vi "Shunting yard algorithm.vi"(2 "error in (no error)":errorcluster, 3 "Infix Notation Data":T1) -> (0 "error out":errorcluster, 1 "Postfix Notation Data":T1)   [LabVIEW 2020]
uses:
  <vilib>/Utility/error.llb/Error Cluster From Error Code.vi
  <vilib>/ErrorRing/Error Ring.xnode
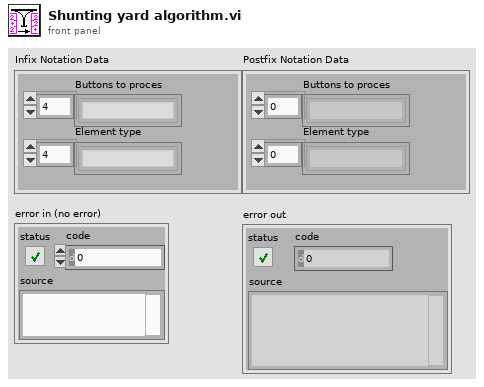
[diagram p1: front panel]
types:
  T1 = cluster{"Buttons to proces":string[], "Element type":string[]}
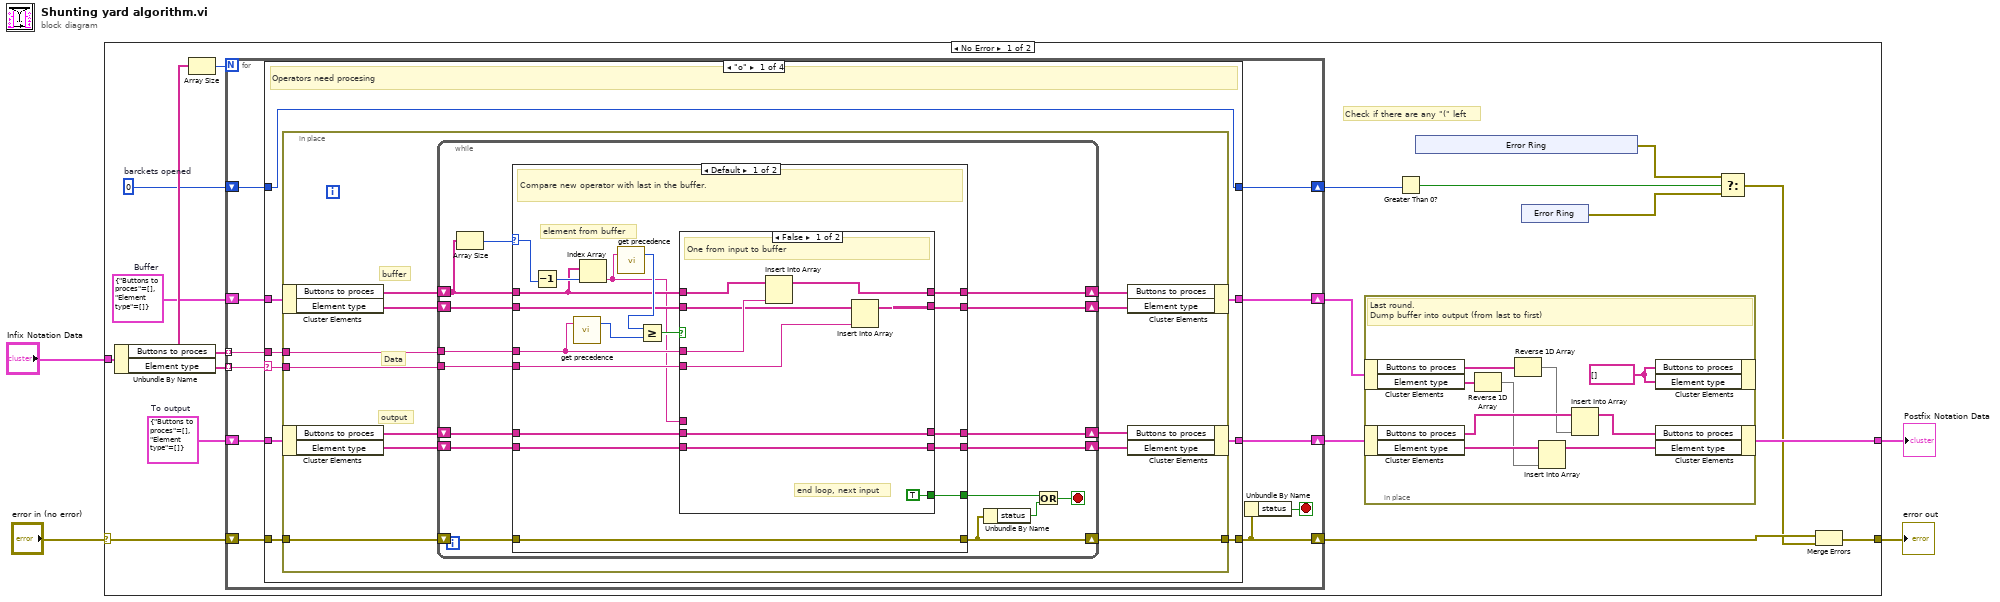
[diagram p0: block diagram]
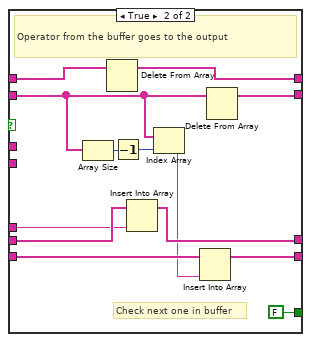
[diagram p2: hidden frame]
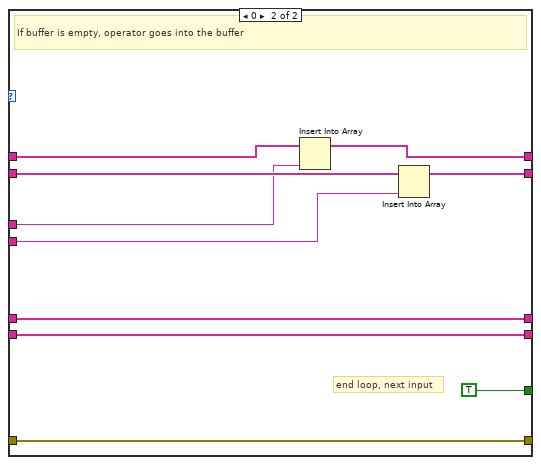
[diagram p3: hidden frame]
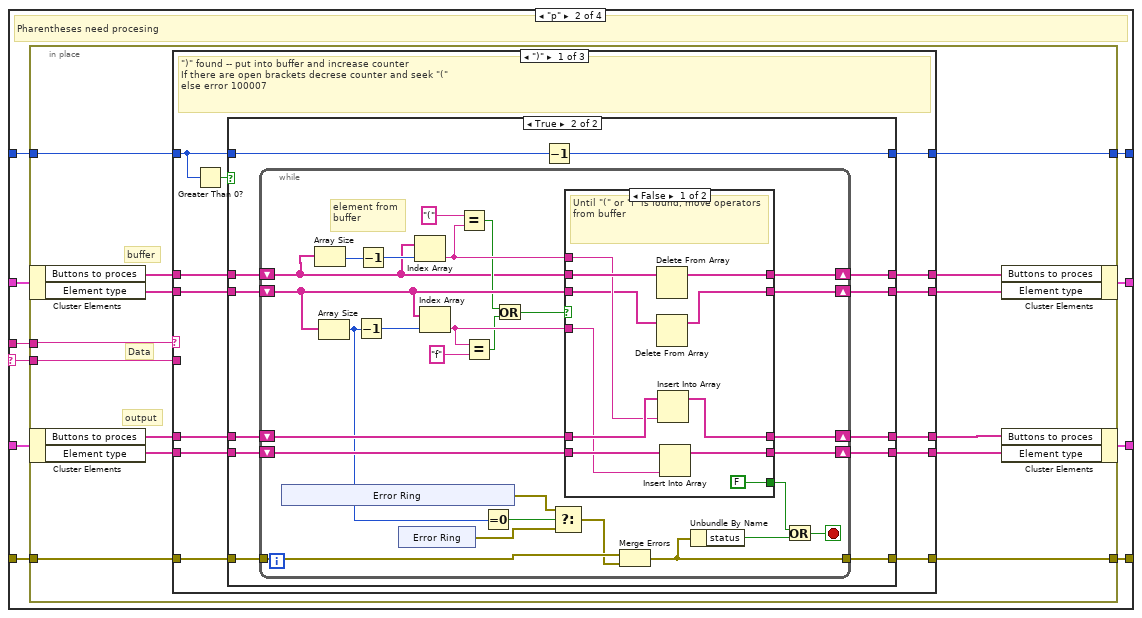
[diagram p4: hidden frame]
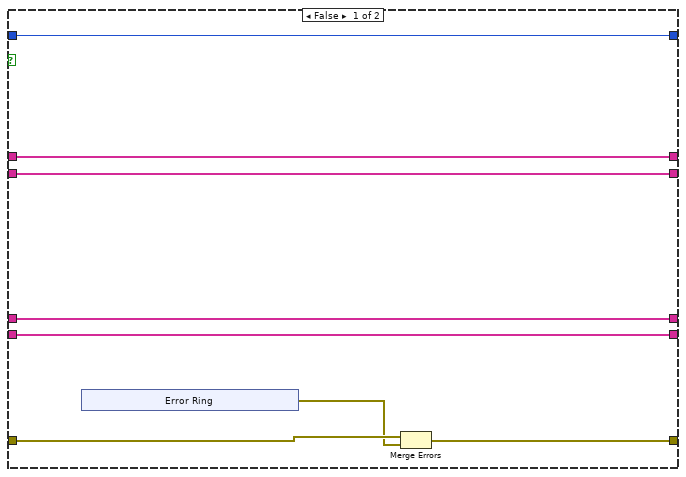
[diagram p5: hidden frame]
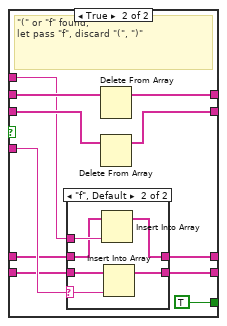
[diagram p6: hidden frame]
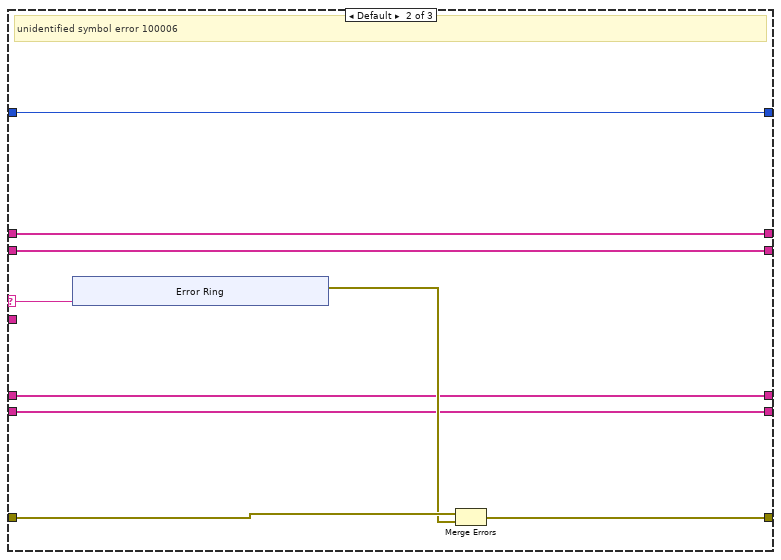
[diagram p8: hidden frame]
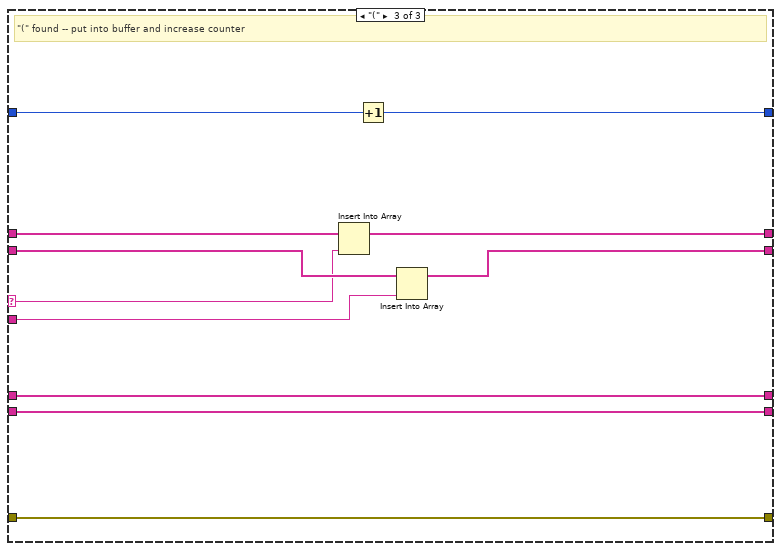
[diagram p9: hidden frame]
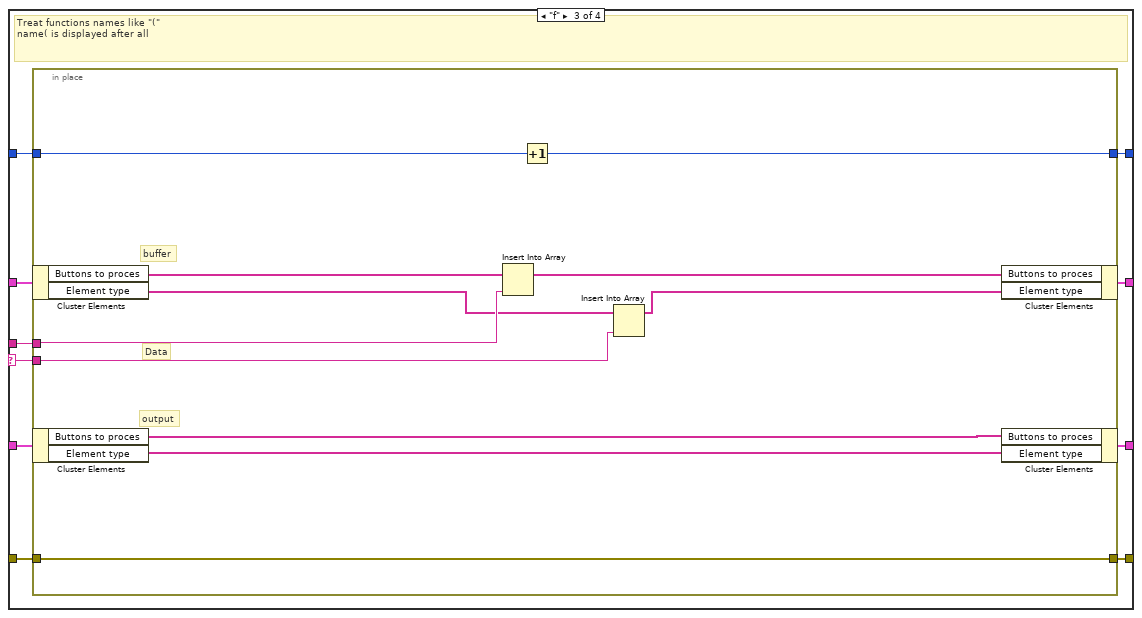
[diagram p10: hidden frame]
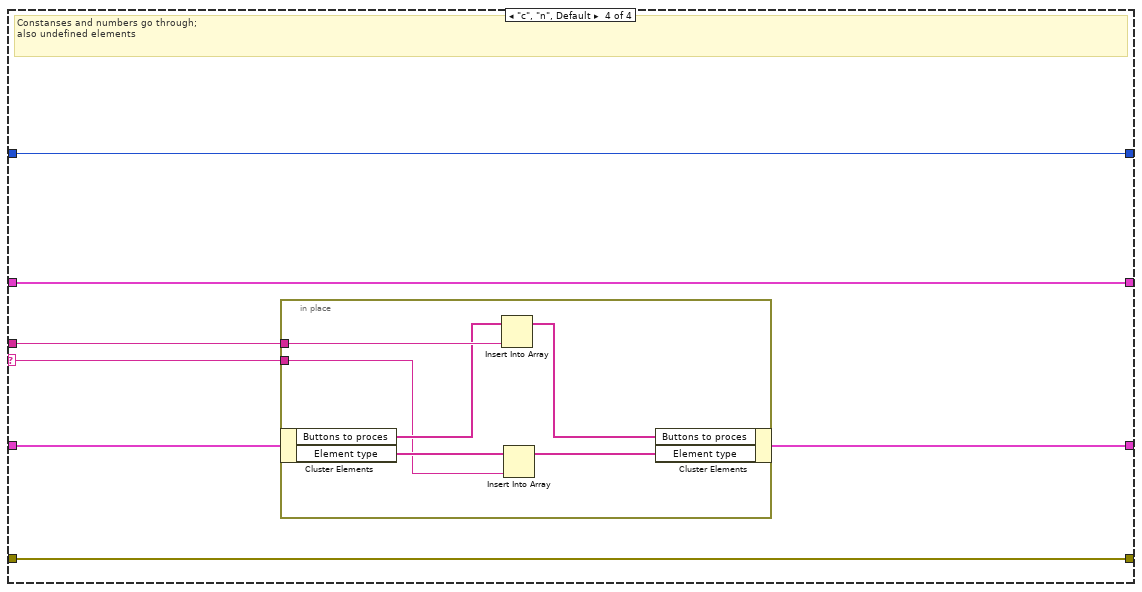
[diagram p11: hidden frame]
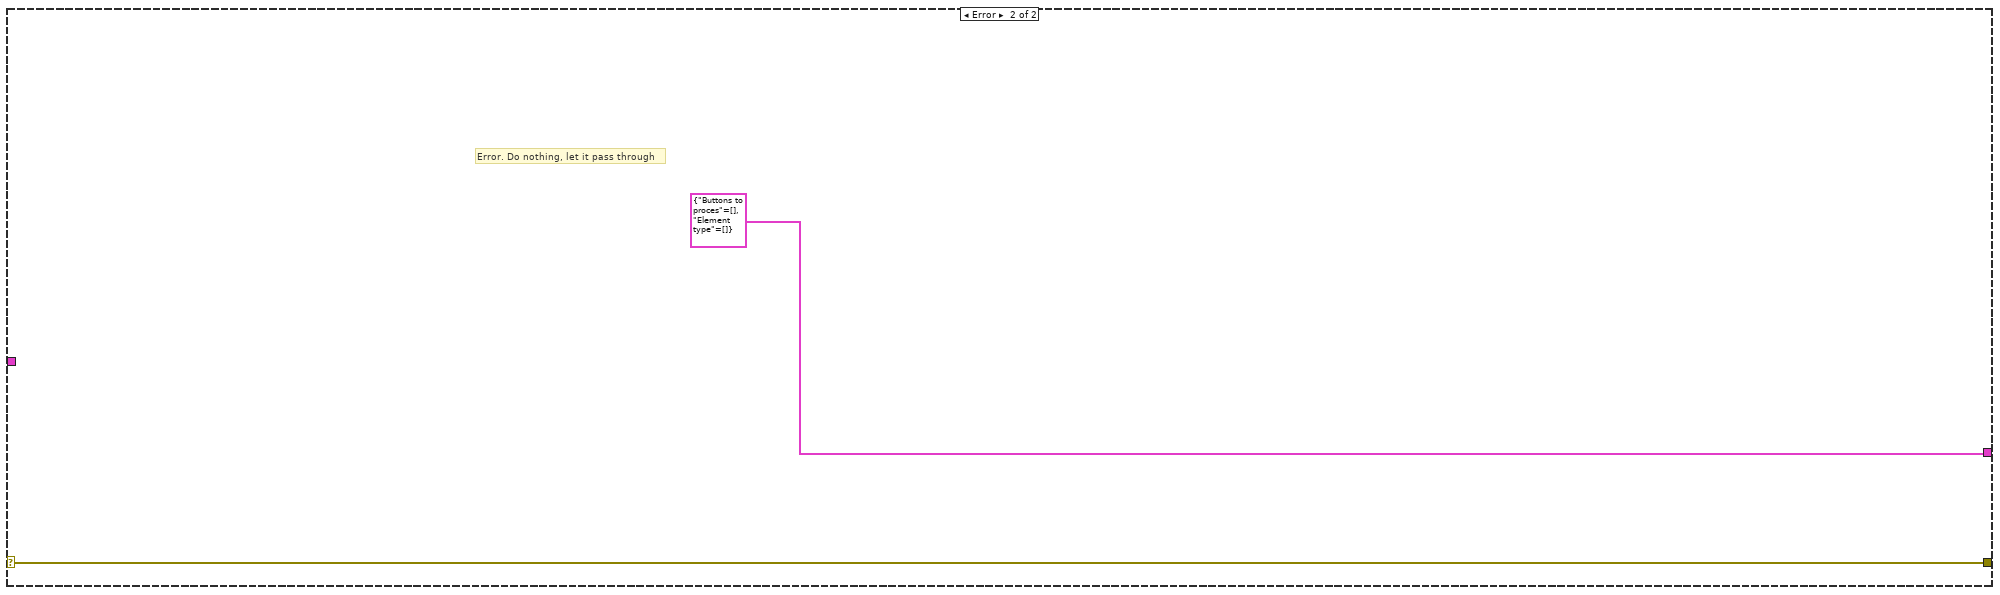
[diagram p12: hidden frame]
diagram:
  n1 = case shown="No Error" "error in (no error)" {
    selector: "error in (no error)" -> [w12 w324]
    tunnel: [w10 w324] -> w3
    tunnel: "Infix Notation Data" -> [w22 _]
    tunnel: [w14 T1 {"Buttons to proces"=[], "Element type"=[]} ("Input Data")] -> w1
    frame No Error {
      w11 = 0  # barckets opened
      w18 = T1 {"Buttons to proces"=[], "Element type"=[]}  # Buffer
      w19 = T1 {"Buttons to proces"=[], "Element type"=[]}  # To output
      # "Check if there are any \"(\" left"
      n2 = Unbundle By Name(w22) -> ("Buttons to proces"=w20:string[], "Element type"=w21:string[])
      n3 = Array Size(array=w20) -> (size(s)=w17:i32)
      n4 = for {
        N: w17 -> [_]
        tunnel: w21 -> [w43] mode=indexing
        tunnel: w20 -> [w44] mode=indexing
        shift-right: [w47] -> w15
        shift-left: w19 -> [w48]
        shift-right: [w45] -> w16
        shift-left: w18 -> [w46]
        shift-right: [w41] -> w13
        shift-left: w12 -> [w42]
        shift-right: [w38] -> w9
        shift-left: w11 -> [w39]
        stop <- w40 stop-if-true
        n5 = case shown="\"o\"" w43 {
          selector: w43 -> [w54 w142 w295 w314]
          tunnel: w48 -> [w57 w145 w298 w316]
          tunnel: [w52 w140 w293 w312] -> w47
          tunnel: w44 -> [w55 w143 w296 w315]
          tunnel: w46 -> [w56 w144 w297 w313]
          tunnel: [w53 w141 w294 w313] -> w45
          tunnel: w42 -> [w51 w139 w292 w311]
          tunnel: [w50 w138 w291 w311] -> w41
          tunnel: w39 -> [w49 w137 w290 w310]
          tunnel: [w49 w136 w289 w310] -> w38
          frame "o" {
            # "Operators need procesing"
            n6 = in-place {
              in-place-border: w55 -> [w63]
              in-place-border: w54 -> [w62]
              in-place-border: w51 -> [w69]
              in-place-border: [w68] -> w50
              # "Data"
              # "buffer"
              # "output"
              n7 = in-place-cluster #1(w56) -> ("Buttons to proces"=w61:string[], "Element type"=w60:string[])
              n8 = in-place-cluster #2(w57) -> ("Buttons to proces"=w65:string[], "Element type"=w64:string[])
              n9 = while {
                shift-right: [w73] -> w68
                shift-left: w69 -> [w74]
                shift-right: [w75] -> w58
                shift-left: w61 -> [w77]
                shift-right: [w78] -> w59
                shift-left: w60 -> [w79]
                shift-right: [w85] -> w67
                shift-left: w65 -> [w83]
                shift-right: [w84] -> w66
                shift-left: w64 -> [w82]
                tunnel: w63 -> [w81]
                tunnel: w62 -> [w80]
                stop <- w70 stop-if-true
                n10 = Array Size(array=w77) -> (size(s)=w76:i32)
                n11 = case shown="Default" w76 {
                  selector: w76 -> [w102 _]
                  tunnel: w83 -> [w94 w129]
                  tunnel: w82 -> [w89 w128]
                  tunnel: w77 -> [w96 w134]
                  tunnel: w79 -> [w98 w132]
                  tunnel: [w90 w128] -> w84
                  tunnel: [w91 w129] -> w85
                  tunnel: w80 -> [w92 w135]
                  tunnel: [w95 w133] -> w75
                  tunnel: [w97 w131] -> w78
                  tunnel: w81 -> [w93 w130]
                  tunnel: w74 -> [w87 w127]
                  tunnel: [w87 w127] -> w73
                  tunnel: [w86 TRUE] -> w71
                  frame Default {
                    # "element from buffer"
                    # "Compare new operator with last in the buffer."
                    n12 = Decrement(x=w102) -> (x-1=w103:i32)
                    n13 = call "get precedence.vi"("operator"=w93) -> ("Precedence"=w100:i32)  [unwired: 2 in]
                    n14 = Index Array(array=w96, index=w103) -> (element=w88:string)
                    n15 = call "get precedence.vi"("operator"=w88) -> ("Precedence"=w101:i32)  [unwired: 2 in]
                    n16 = Greater Or Equal?(x=w101, y=w100) -> (x >= y?=w99:bool)
                    n17 = case shown="False" w99 {
                      tunnel: w98 -> [w107 w115]
                      tunnel: [w104 w124] -> w97
                      tunnel: w96 -> [w106 w118]
                      tunnel: [w105 w125] -> w95
                      tunnel: w94 -> [w109 w123]
                      tunnel: w89 -> [w108 w122]
                      tunnel: w93 -> [w112 _]
                      tunnel: w92 -> [w111 _]
                      tunnel: [w108 w121] -> w90
                      tunnel: [w109 w119] -> w91
                      tunnel: w88 -> [_ w120]
                      tunnel: [TRUE FALSE] -> w86
                      frame False {
                        # "end loop, next input"
                        # "One from input to buffer"
                        n18 = Insert Into Array(array=w106, new element=w112) -> (w105:string[])  [unwired: 1 in]
                        n19 = Insert Into Array(array=w107, new element=w111) -> (w104:string[])  [unwired: 1 in]
                      }
                      frame True {
                        # "Check next one in buffer"
                        # "Operator from the buffer goes to the output"
                        n20 = Array Size(array=w115) -> (size(s)=w117:i32)
                        n21 = Delete From Array(array=w118) -> (array with subset deleted=w125:string[])  [unwired: 2 in, 1 out]
                        n22 = Decrement(x=w117) -> (x-1=w116:i32)
                        n23 = Insert Into Array(array=w123, new element=w120) -> (w119:string[])  [unwired: 1 in]
                        n24 = Index Array(array=w115, index=w116) -> (element=w114:string)
                        n25 = Insert Into Array(array=w122, new element=w114) -> (w121:string[])  [unwired: 1 in]
                        n26 = Delete From Array(array=w115) -> (array with subset deleted=w124:string[])  [unwired: 2 in, 1 out]
                      }
                    }
                  }
                  frame 0 {
                    # "end loop, next input"
                    # "If buffer is empty, operator goes into the buffer"
                    n27 = Insert Into Array(array=w134, new element=w130) -> (w133:string[])  [unwired: 1 in]
                    n28 = Insert Into Array(array=w132, new element=w135) -> (w131:string[])  [unwired: 1 in]
                  }
                }
                n29 = Unbundle By Name(w73) -> ("status"=w72:bool)
                n30 = Or(x=w71, y=w72) -> (x .or. y?=w70:bool)
              }
              n31 = in-place-cluster #1("Buttons to proces"=w58, "Element type"=w59) -> (w53:T1)
              n32 = in-place-cluster #2("Buttons to proces"=w67, "Element type"=w66) -> (w52:T1)
            }
          }
          frame "p" {
            # "Pharentheses need procesing"
            n33 = in-place {
              in-place-border: w143 -> [w159]
              in-place-border: w142 -> [w148]
              in-place-border: w139 -> [w158]
              in-place-border: [w157] -> w138
              in-place-border: w137 -> [w146]
              in-place-border: [w147] -> w136
              # "Data"
              # "buffer"
              # "output"
              n34 = in-place-cluster #3(w144) -> ("Buttons to proces"=w155:string[], "Element type"=w154:string[])
              n35 = in-place-cluster #4(w145) -> ("Buttons to proces"=w151:string[], "Element type"=w149:string[])
              n36 = case shown="\")\"" w159 {
                selector: w159 -> [_ w270 w282]
                tunnel: w158 -> [w169 w268 w280]
                tunnel: [w168 w269 w280] -> w157
                tunnel: [w166 w266 w285] -> w156
                tunnel: w155 -> [w167 w266 w286]
                tunnel: w154 -> [w165 w265 w284]
                tunnel: [w164 w265 w283] -> w153
                tunnel: [w163 w264 w288] -> w152
                tunnel: w151 -> [w162 w264 w288]
                tunnel: [w161 w263 w287] -> w150
                tunnel: w149 -> [w160 w263 w287]
                tunnel: w148 -> [_ _ w281]
                tunnel: [w170 w262 w278] -> w147
                tunnel: w146 -> [w171 w262 w279]
                frame ")" {
                  # "\")\" found -- put into buffer and increase counter\nIf there are open brackets decrese counter and seek \"(\"\nelse error 100007"
                  n37 = Greater Than 0?(x=w171) -> (x > 0?=w172:bool)
                  n38 = case shown="True" w172 {
                    tunnel: w171 -> [w180 w197]
                    tunnel: [w180 w196] -> w170
                    tunnel: w169 -> [w178 w194]
                    tunnel: [w179 w195] -> w168
                    tunnel: w167 -> [w177 w186]
                    tunnel: [w177 w193] -> w166
                    tunnel: w165 -> [w176 w192]
                    tunnel: [w176 w191] -> w164
                    tunnel: [w175 w188] -> w163
                    tunnel: w162 -> [w175 w190]
                    tunnel: [w174 w187] -> w161
                    tunnel: w160 -> [w174 w189]
                    frame False {
                      n39 = xnode "Error Ring"() -> ("error out"=w173:errorcluster)
                      n40 = Merge Errors(w178, w173) -> (w179:errorcluster)
                    }
                    frame True {
                      n41 = while {
                        tunnel: [w198] -> w195
                        tunnel: w194 -> [w217]
                        shift-right: [w224] -> w193
                        shift-left: w186 -> [w206]
                        shift-right: [w223] -> w191
                        shift-left: w192 -> [w222]
                        shift-right: [w221] -> w188
                        shift-left: w190 -> [w220]
                        shift-right: [w219] -> w187
                        shift-left: w189 -> [w218]
                        stop <- w216 stop-if-true
                        # "element from buffer"
                        n42 = xnode "Error Ring"() -> ("error out"=w199:errorcluster)
                        n43 = Array Size(array=w206) -> (size(s)=w205:i32)
                        n44 = Array Size(array=w222) -> (size(s)=w202:i32)
                        n45 = Decrement(x=w202) -> (x-1=w213:i32)
                        n46 = Decrement(x=w205) -> (x-1=w225:i32)
                        n47 = xnode "Error Ring"() -> ("error out"=w201:errorcluster)
                        n48 = Index Array(array=w206, index=w225) -> (element=w212:string)
                        n49 = Index Array(array=w222, index=w213) -> (element=w210:string)
                        n50 = Equal?(x="(", y=w212) -> (x = y?=w211:bool)
                        n51 = Equal?(x=w210, y="f") -> (x = y?=w209:bool)
                        n52 = Equal To 0?(x=w202) -> (x = 0?=w203:bool)
                        n53 = Or(x=w211, y=w209) -> (x .or. y?=w214:bool)
                        n54 = Select(t=w199, s=w203, f=w201) -> (s? t:f=w200:errorcluster)
                        n55 = case shown="False" w214 {
                          tunnel: w206 -> [w242 w253]
                          tunnel: [w241 w252] -> w224
                          tunnel: [w240 w250] -> w223
                          tunnel: w222 -> [w234 w251]
                          tunnel: [w236 w247] -> w221
                          tunnel: w220 -> [w237 w246]
                          tunnel: [w239 w245] -> w219
                          tunnel: w218 -> [w238 w244]
                          tunnel: [FALSE TRUE] -> w215
                          tunnel: w212 -> [w235 w243]
                          tunnel: w210 -> [w233 w248]
                          frame False {
                            # "Until \"(\" or \"f\" is found, move operators from buffer"
                            n56 = Delete From Array(array=w242) -> (array with subset deleted=w241:string[])  [unwired: 2 in, 1 out]
                            n57 = Delete From Array(array=w234) -> (array with subset deleted=w240:string[])  [unwired: 2 in, 1 out]
                            n58 = Insert Into Array(array=w237, new element=w235) -> (w236:string[])  [unwired: 1 in]
                            n59 = Insert Into Array(array=w238, new element=w233) -> (w239:string[])  [unwired: 1 in]
                          }
                          frame True {
                            # "\"(\" or \"f\" found,\nlet pass \"f\", discard \"(\", \")\""
                            n60 = case shown="\"f\", Default" w248 {
                              selector: w248 -> [_ w259]
                              tunnel: [w255 w256] -> w247
                              tunnel: w246 -> [w255 w257]
                              tunnel: [w254 w260] -> w245
                              tunnel: w244 -> [w254 w261]
                              tunnel: w243 -> [_ w258]
                              frame "p" {
                              }
                              frame "f", Default {
                                n61 = Insert Into Array(array=w257, new element=w258) -> (w256:string[])  [unwired: 1 in]
                                n62 = Insert Into Array(array=w261, new element=w259) -> (w260:string[])  [unwired: 1 in]
                              }
                            }
                            n63 = Delete From Array(array=w253) -> (array with subset deleted=w252:string[])  [unwired: 2 in, 1 out]
                            n64 = Delete From Array(array=w251) -> (array with subset deleted=w250:string[])  [unwired: 2 in, 1 out]
                          }
                        }
                        n65 = Merge Errors(w217, w200) -> (w198:errorcluster)
                        n66 = Unbundle By Name(w198) -> ("status"=w204:bool)
                        n67 = Or(x=w215, y=w204) -> (x .or. y?=w216:bool)
                      }
                      n68 = Decrement(x=w197) -> (x-1=w196:i32)
                    }
                  }
                }
                frame Default {
                  # "unidentified symbol error 100006"
                  n69 = xnode "Error Ring"("parameter 0"=w270) -> ("error out"=w267:errorcluster)
                  n70 = Merge Errors(w268, w267) -> (w269:errorcluster)
                }
                frame "(" {
                  # "\"(\" found -- put into buffer and increase counter"
                  n71 = Insert Into Array(array=w286, new element=w282) -> (w285:string[])  [unwired: 1 in]
                  n72 = Increment(x=w279) -> (x+1=w278:i32)
                  n73 = Insert Into Array(array=w284, new element=w281) -> (w283:string[])  [unwired: 1 in]
                }
              }
              n74 = in-place-cluster #3("Buttons to proces"=w156, "Element type"=w153) -> (w141:T1)
              n75 = in-place-cluster #4("Buttons to proces"=w152, "Element type"=w150) -> (w140:T1)
            }
          }
          frame "f" {
            # "Treat functions names like \"(\"\nname( is displayed after all"
            n76 = in-place {
              in-place-border: w296 -> [w309]
              in-place-border: w295 -> [w301]
              in-place-border: w292 -> [w308]
              in-place-border: [w308] -> w291
              in-place-border: w290 -> [w299]
              in-place-border: [w300] -> w289
              # "Data"
              # "buffer"
              # "output"
              n77 = in-place-cluster #5(w297) -> ("Buttons to proces"=w306:string[], "Element type"=w305:string[])
              n78 = in-place-cluster #6(w298) -> ("Buttons to proces"=w303:string[], "Element type"=w302:string[])
              n79 = Insert Into Array(array=w306, new element=w309) -> (w307:string[])  [unwired: 1 in]
              n80 = Increment(x=w299) -> (x+1=w300:i32)
              n81 = Insert Into Array(array=w305, new element=w301) -> (w304:string[])  [unwired: 1 in]
              n82 = in-place-cluster #5("Buttons to proces"=w307, "Element type"=w304) -> (w294:T1)
              n83 = in-place-cluster #6("Buttons to proces"=w303, "Element type"=w302) -> (w293:T1)
            }
          }
          frame "c", "n", Default {
            # "Constanses and numbers go through;\nalso undefined elements"
            n84 = in-place {
              in-place-border: w315 -> [w322]
              in-place-border: w314 -> [w317]
              n85 = in-place-cluster #7(w316) -> ("Buttons to proces"=w321:string[], "Element type"=w319:string[])
              n86 = Insert Into Array(array=w321, new element=w322) -> (w320:string[])  [unwired: 1 in]
              n87 = Insert Into Array(array=w319, new element=w317) -> (w318:string[])  [unwired: 1 in]
              n88 = in-place-cluster #7("Buttons to proces"=w320, "Element type"=w318) -> (w312:T1)
            }
          }
        }
        n89 = Unbundle By Name(w41) -> ("status"=w40:bool)
      }
      n90 = in-place {
        w29 = string[] [] ("Buttons to proces")
        # "Last round.\nDump buffer into output (from last to first)"
        n91 = in-place-cluster #8(w16) -> ("Buttons to proces"=w33:string[], "Element type"=w32:string[])
        n92 = in-place-cluster #9(w15) -> ("Buttons to proces"=w37:string[], "Element type"=w34:string[])
        n93 = Reverse 1D Array(array=w32) -> (reversed array=w31:string[])
        n94 = Reverse 1D Array(array=w33) -> (reversed array=w30:string[])
        n95 = Insert Into Array(array=w34, new element=w31) -> (w35:string[])  [unwired: 1 in]
        n96 = Insert Into Array(array=w37, new element=w30) -> (w36:string[])  [unwired: 1 in]
        n97 = in-place-cluster #8("Buttons to proces"=w29, "Element type"=w29) -> ()  [unwired: 1 out]
        n98 = in-place-cluster #9("Buttons to proces"=w36, "Element type"=w35) -> (w14:T1)
      }
      n99 = Greater Than 0?(x=w9) -> (x > 0?=w8:bool)
      n100 = xnode "Error Ring"() -> ("error out"=w6:errorcluster)
      n101 = xnode "Error Ring"() -> ("error out"=w5:errorcluster)
      n102 = Select(t=w6, s=w8, f=w5) -> (s? t:f=w7:errorcluster)
      n103 = Merge Errors(w13, w7) -> (w10:errorcluster)
    }
    frame Error {
      # "Error. Do nothing, let it pass through"
    }
  }
  "Postfix Notation Data" <- w1
  "error out" <- w3
